vi "ATM_Serv.vi"() -> ()   [LabVIEW 2023]
uses:
  Controller/ControllerATM.ctl
  Controller/ControllerMenu.ctl
  Controller/ControllerAccount.ctl
  <vilib>/Utility/file.llb/Read Delimited Spreadsheet (string).vi
  <vilib>/Utility/file.llb/Write Delimited Spreadsheet (string).vi
  <vilib>/regexp/Match Regular Expression.xnode
panel:
  out "event error":errorcluster
  out "Output":string
  out "login error":errorcluster
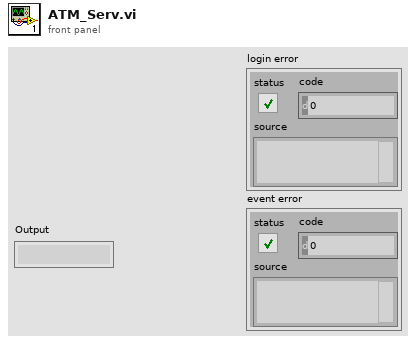
[diagram p1: front panel]
types:
  T1 = typedef "ControllerAccount.ctl" = enum16{"Deactivate", "Deposit", "Withdraw"}
  T2 = typedef "ControllerMenu.ctl" = enum16{"Initialization", "Processes"}
  T3 = typedef "ControllerATM.ctl" = enum16{"Welcome", "Login", "Main"}
  T4 = enum16{"open", "replace", "create", "open or create", "replace or create", "replace or create with confirmation"}
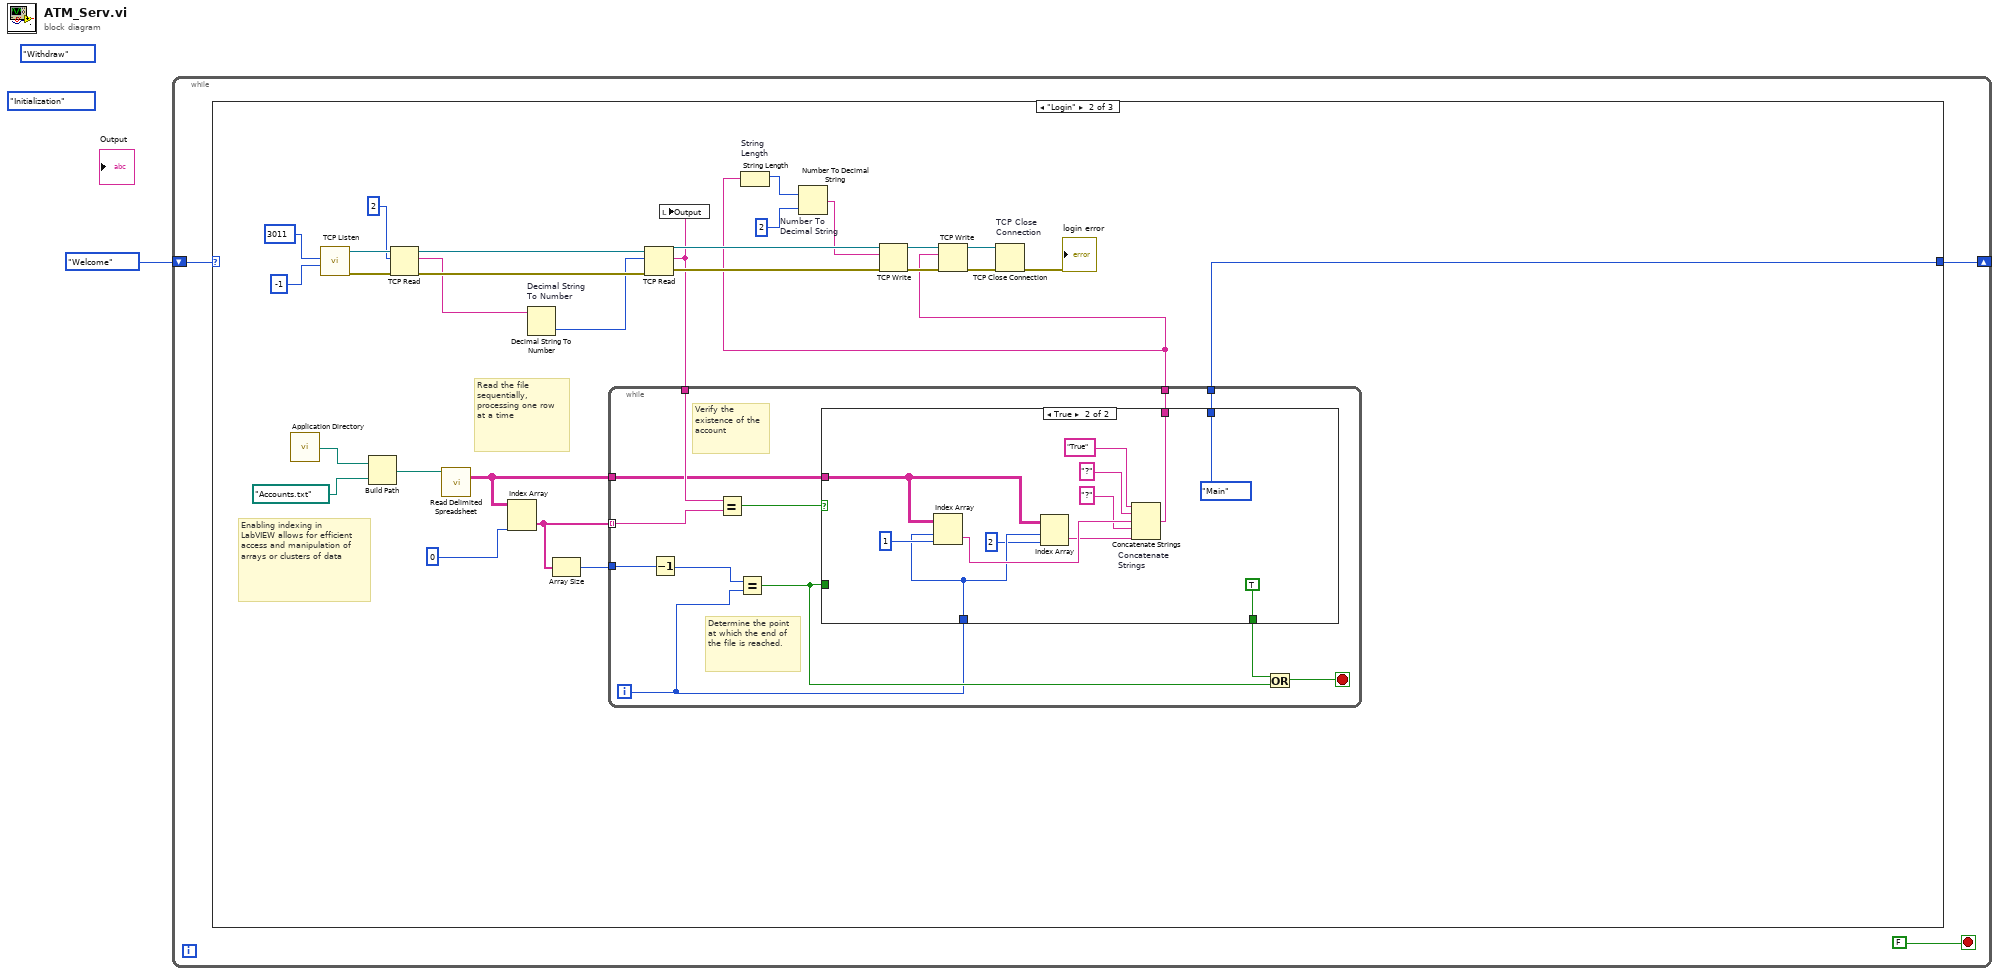
[diagram p0: block diagram]
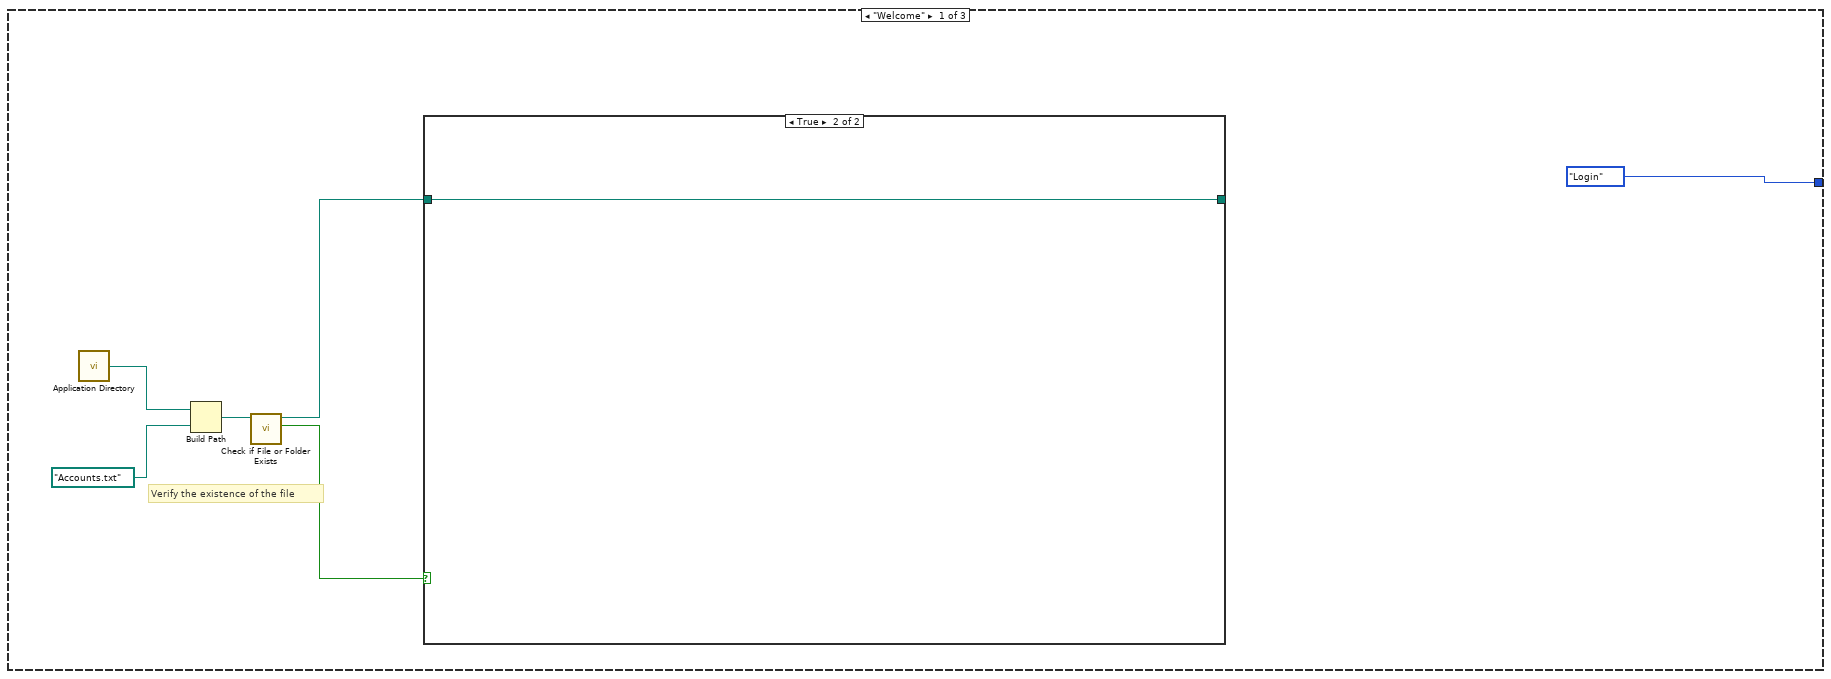
[diagram p2: hidden frame]
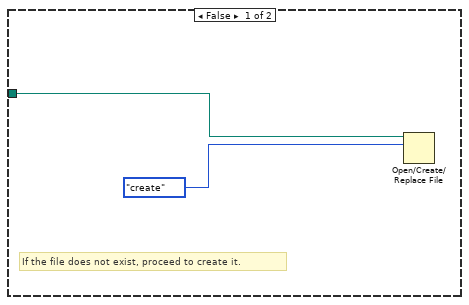
[diagram p3: hidden frame]
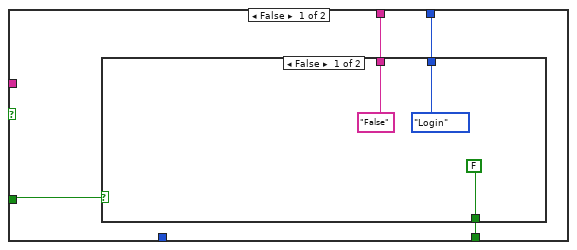
[diagram p4: hidden frame]
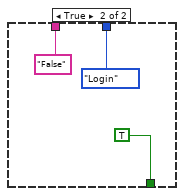
[diagram p5: hidden frame]
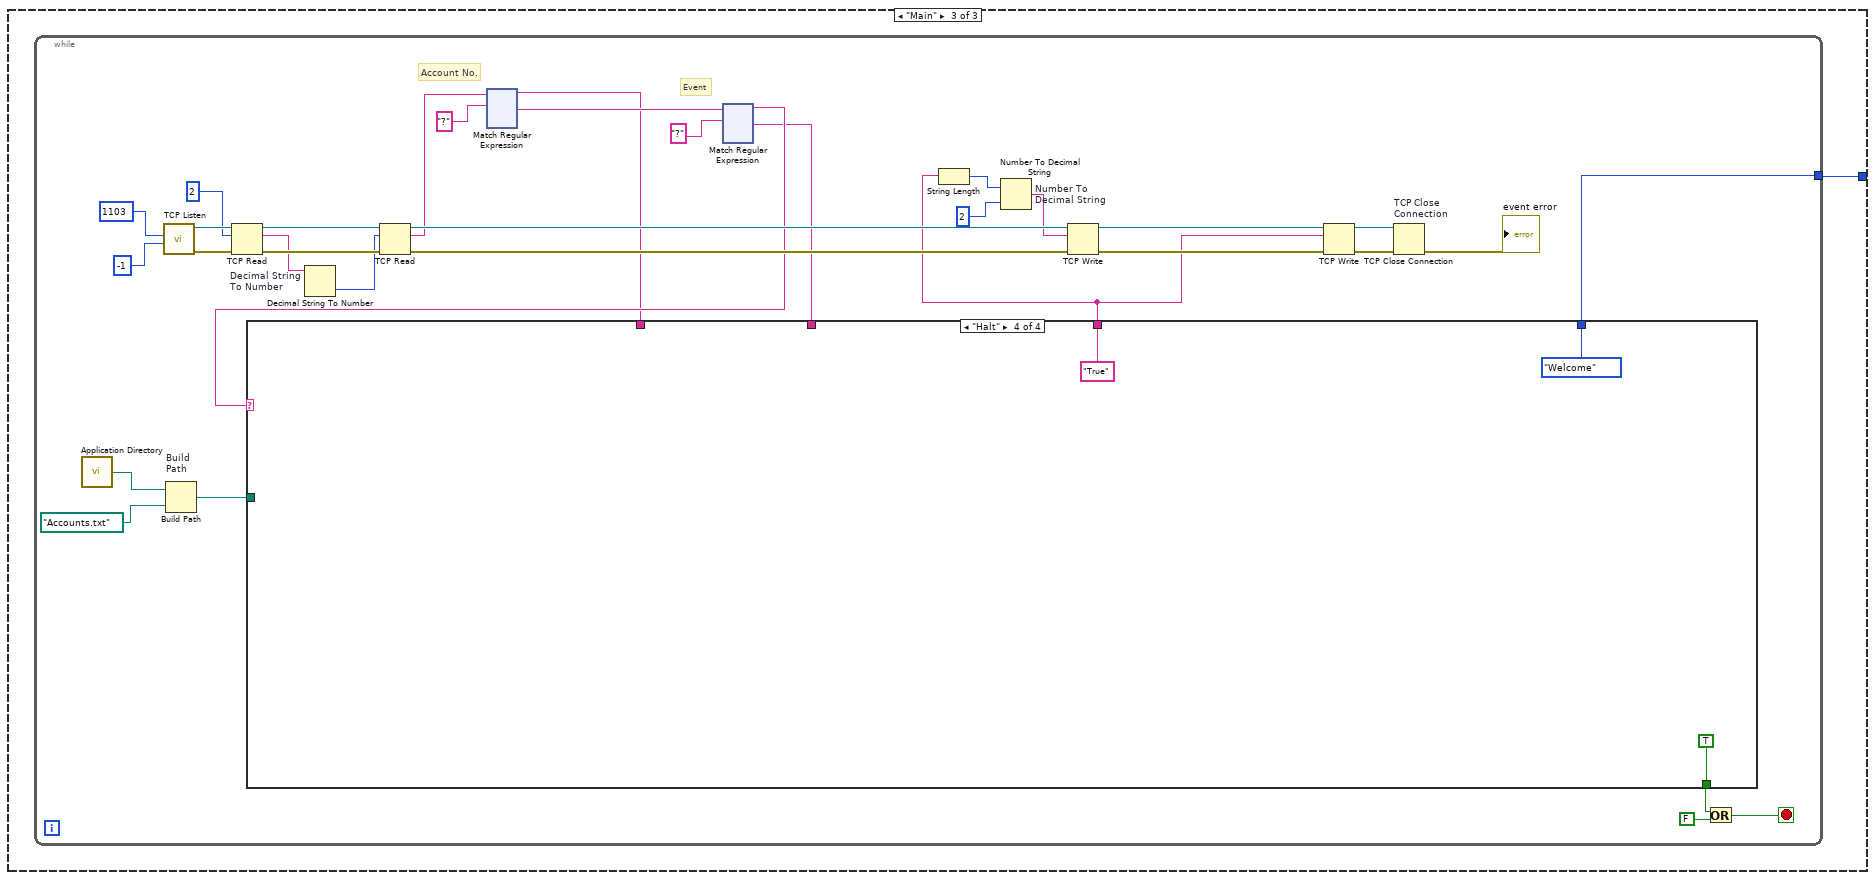
[diagram p6: hidden frame]
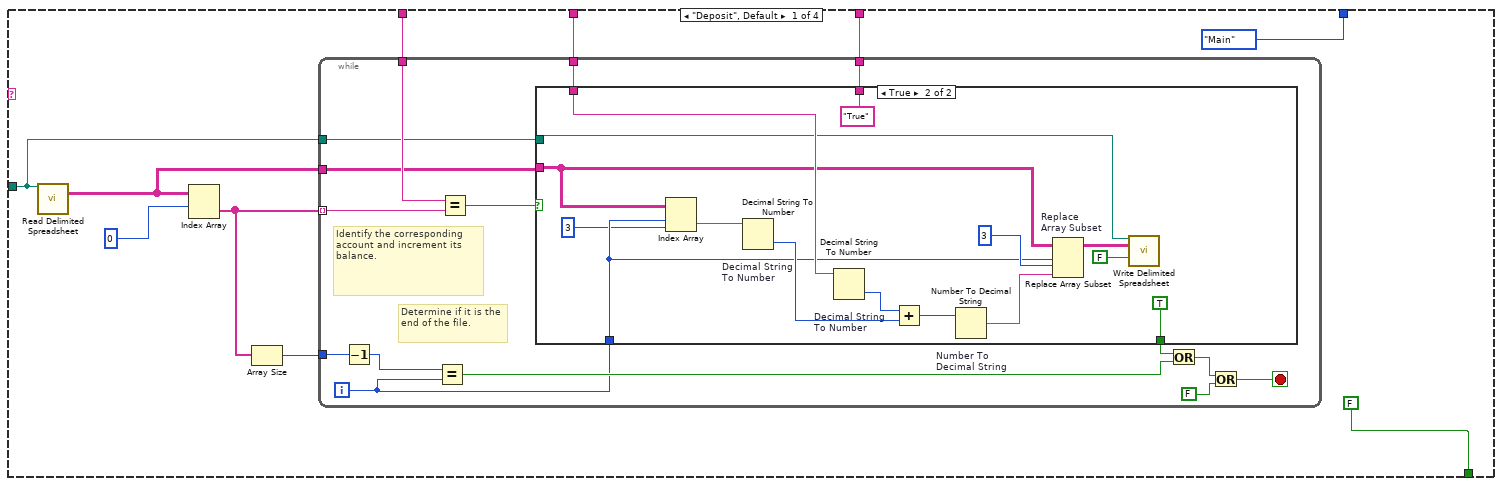
[diagram p7: hidden frame]
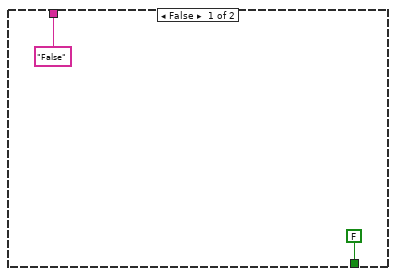
[diagram p8: hidden frame]
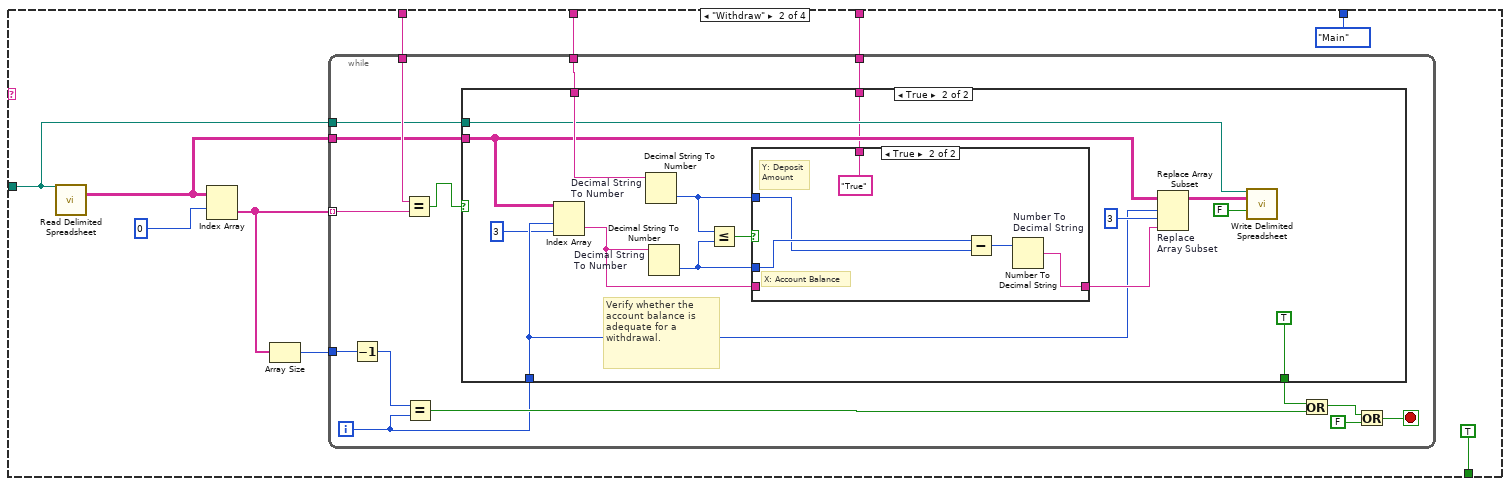
[diagram p9: hidden frame]
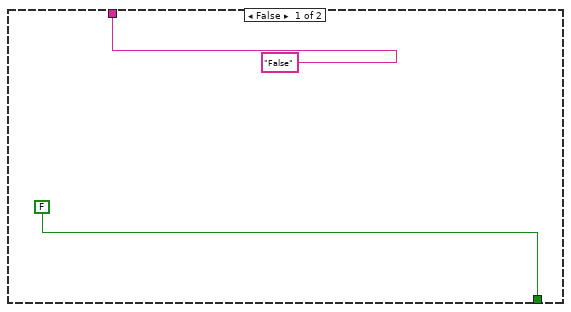
[diagram p10: hidden frame]
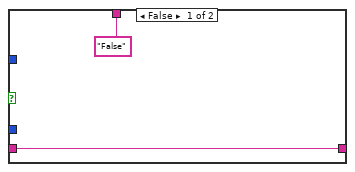
[diagram p11: hidden frame]
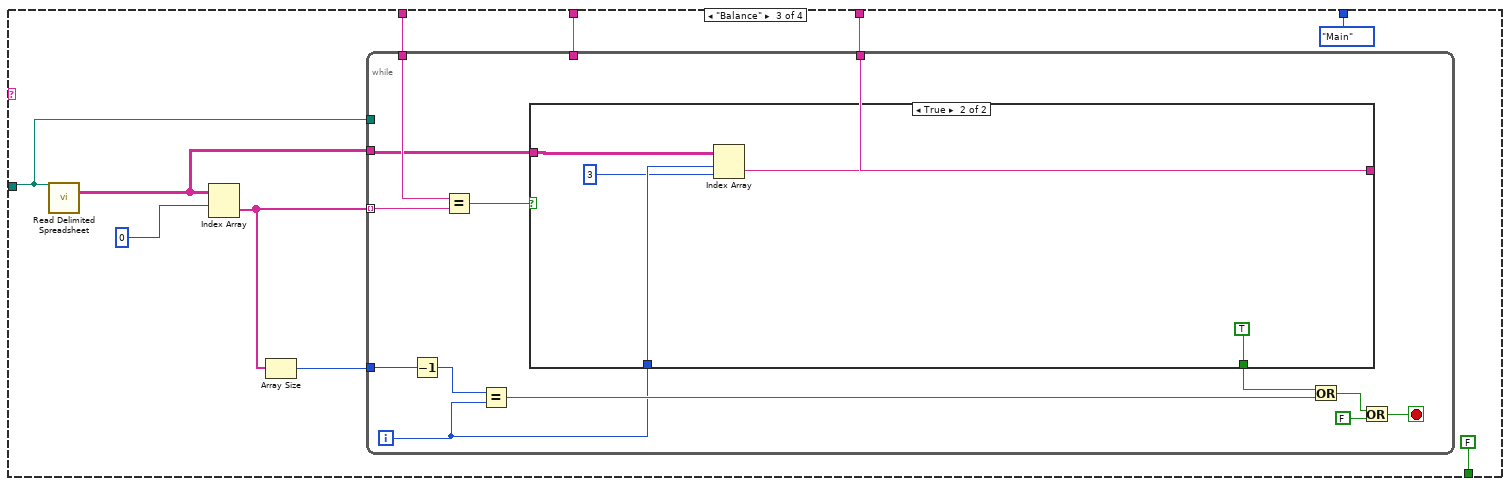
[diagram p12: hidden frame]
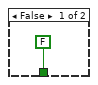
[diagram p13: hidden frame]
diagram:
  (unwired) ControllerAccount."Withdraw" ("Enter")
  (unwired) ControllerMenu."Initialization"
  n1 = while {
    shift-right: [w2] -> _
    shift-left: ControllerATM."Welcome" -> [w3]
    stop <- FALSE stop-if-true
    n2 = case shown="\"Login\"" w3 {
      tunnel: [ControllerATM."Login" w15 w77] -> w2
      frame "Welcome" {
        # "Verify the existence of the file"
        n3 = call <vilib>:"Application Directory.vi"() -> ("Application Directory"=w9:path)
        n4 = Build Path(base path=w9, name or relative path=path "Accounts.txt") -> (appended path=w7:path)
        n5 = call <vilib>:"Check if File or Folder Exists.vi"("path"=w7) -> ("file or folder exists?"=w8:bool, "dup path"=w6:path)  [unwired: 8 in, 1 out]
        n6 = case shown="True" w8 {
          tunnel: w6 -> [w11 w13]
          tunnel: [_ w13] -> _
          frame False {
            # "If the file does not exist, proceed to create it."
            n7 = Open/Create/Replace File(file path (use dialog)=w11, operation (0:open)=T4."create") -> ()  [unwired: 4 in, 3 out]
          }
          frame True {
          }
        }
      }
      frame "Login" {
        # "Enabling indexing in LabVIEW allows for efficient access and manipulation of arrays or clusters of data"
        # "Read the file sequentially, processing one row at a time"
        n8 = call <vilib>:"Application Directory.vi"() -> ("Application Directory"=w22:path)
        n9 = call <vilib>:"TCP Listen.vi"("timeout ms (wait forever: -1)"=-1, "port"=u16 3011) -> ("error out"=w38:errorcluster, "connection ID"=w42:refnum<k5>)  [unwired: 5 in, 3 out]
        n10 = Build Path(base path=w22, name or relative path=path "Accounts.txt") -> (appended path=w23:path)
        n11 = TCP Read(connection ID=w42, bytes to read=2, error in (no error)=w38) -> (connection ID out=w41:refnum<k5>, data out=w29:string, error out=w37:errorcluster)  [unwired: 2 in]
        n12 = call-poly <vilib>:"Read Delimited Spreadsheet.vi"("file path (dialog if empty)"=w23) -> ("all rows"=w20:string[][])  [unwired: 9 in, 5 out]
        n13 = Index Array "Index Array"(array=w20, index (col)=0 ("index (row)")) -> (element=w19:string[])  [unwired: 1 in]
        n14 = Decimal String To Number "Decimal String \nTo Number"(string=w29) -> (number=w28:i32)  [unwired: 2 in, 1 out]
        n15 = Array Size(array=w19) -> (size(s)=w18:i32)
        n16 = TCP Read(connection ID=w41, bytes to read=w28, error in (no error)=w37) -> (connection ID out=w40:refnum<k5>, data out=w24:string, error out=w36:errorcluster)  [unwired: 2 in]
        n17 = while {
          tunnel: w24 -> [w49]
          tunnel: w19 -> [w48] mode=indexing
          tunnel: w20 -> [w46]
          tunnel: w18 -> [w54]
          tunnel: [w44] -> w16
          tunnel: [w43] -> w15
          i -> [w45]
          stop <- w51 stop-if-true
          # "Determine the point at which the end of the file is reached."
          # "Verify the existence of the account"
          n18 = Decrement(x=w54) -> (x-1=w53:i32)
          n19 = Equal?(x=w49, y=w48) -> (x = y?=w47:bool)
          n20 = Equal?(x=w53, y=w45) -> (x = y?=w50:bool)
          n21 = case shown="True" w47 {
            tunnel: w50 -> [w58 _]
            tunnel: [w56 TRUE] -> w52
            tunnel: w46 -> [_ w75]
            tunnel: w45 -> [_ w67]
            tunnel: [w57 w69] -> w44
            tunnel: [w55 ControllerATM."Main"] -> w43
            frame False {
              n22 = case shown="False" w58 {
                tunnel: ["False" "False"] -> w57
                tunnel: [ControllerATM."Login" ControllerATM."Login"] -> w55
                tunnel: [FALSE TRUE] -> w56
                frame False {
                }
                frame True {
                }
              }
            }
            frame True {
              n23 = Index Array "Index Array"(array=w75, index (row)=w67, index (col)=1 ("index (row)")) -> (element=w72:string)
              n24 = Index Array "Index Array"(array=w75, index (row)=w67, index (col)=2 ("index (row)")) -> (element=w70:string)
              n25 = Concatenate Strings "Concatenate\nStrings"("True" ("string"), "?" ("string"), w72, "?" ("string"), w70) -> (w69:string)
            }
          }
          n26 = Or(x=w52, y=w50) -> (x .or. y?=w51:bool)
        }
        n27 = local write "Output"(w24) -> ()
        n28 = String Length "String \nLength"(string=w16) -> (length=w25:i32)
        n29 = Number To Decimal String "Number To \nDecimal String"(number=w25, width (-)=i16 2) -> (decimal integer string=w27:string)
        n30 = TCP Write(connection ID=w40, data in=w27, error in (no error)=w36) -> (connection ID out=w17:refnum<k5>, error out=w35:errorcluster)  [unwired: 1 in, 1 out]
        n31 = TCP Write(connection ID=w17, data in=w16, error in (no error)=w35) -> (connection ID out=w39:refnum<k5>, error out=w34:errorcluster)  [unwired: 1 in, 1 out]
        n32 = TCP Close Connection "TCP Close \nConnection"(connection ID=w39, error in (no error)=w34) -> (error out=→"login error":errorcluster)  [unwired: 1 in, 1 out]
      }
      frame "Main" {
        n33 = while {
          tunnel: [w81] -> w77
          stop <- w80 stop-if-true
          # "Event"
          # "Account No."
          n34 = call <vilib>:"Application Directory.vi"() -> ("Application Directory"=w88:path)
          n35 = call <vilib>:"TCP Listen.vi"("timeout ms (wait forever: -1)"=-1, "port"=u16 1103) -> ("error out"=w106:errorcluster, "connection ID"=w111:refnum<k5>)  [unwired: 5 in, 3 out]
          n36 = Build Path "Build\nPath"(base path=w88, name or relative path=path "Accounts.txt") -> (appended path=w84:path)
          n37 = TCP Read(connection ID=w111, bytes to read=2, error in (no error)=w106) -> (connection ID out=w110:refnum<k5>, data out=w97:string, error out=w105:errorcluster)  [unwired: 2 in]
          n38 = Decimal String To Number "Decimal String\nTo Number"(string=w97) -> (number=w96:i32)  [unwired: 2 in, 1 out]
          n39 = TCP Read(connection ID=w110, bytes to read=w96, error in (no error)=w105) -> (connection ID out=w109:refnum<k5>, data out=w95:string, error out=w104:errorcluster)  [unwired: 2 in]
          n40 = xnode "Match Regular \nExpression"("input string"=w95, "regular expression"="?") -> ("before match"=w85:string, "after match"=w93:string)  [unwired: 4 in, 3 out]
          n41 = xnode "Match Regular \nExpression"("input string"=w93, "regular expression"="?") -> ("before match"=w86:string, "after match"=w83:string)  [unwired: 4 in, 3 out]
          n42 = case shown="\"Halt\"" w86 {
            tunnel: w84 -> [w112 w157 w208 _]
            tunnel: w85 -> [w118 w156 w207 _]
            tunnel: w83 -> [w116 w155 w206 _]
            tunnel: [w115 w154 w205 "True"] -> w82
            tunnel: [ControllerATM."Main" ControllerATM."Main" ControllerATM."Main" ControllerATM."Welcome"] -> w81
            tunnel: [FALSE ("x") TRUE ("x") FALSE ("x") TRUE ("x")] -> w78
            frame "Deposit", Default {
              n43 = call-poly <vilib>:"Read Delimited Spreadsheet.vi"("file path (dialog if empty)"=w112) -> ("all rows"=w117:string[][])  [unwired: 9 in, 5 out]
              n44 = Index Array "Index Array"(array=w117, index (row)=0 ("index")) -> (element=w119:string[])  [unwired: 1 in]
              n45 = Array Size(array=w119) -> (size(s)=w120:i32)
              n46 = while {
                tunnel: w120 -> [w131]
                tunnel: w119 -> [w129] mode=indexing
                tunnel: w118 -> [w128]
                tunnel: w117 -> [w125]
                tunnel: w112 -> [w123]
                tunnel: w116 -> [w124]
                tunnel: [w122] -> w115
                i -> [w126]
                stop <- w136 stop-if-true
                # "Determine if it is the end of the file."
                # "Identify the corresponding account and increment its balance."
                n47 = Decrement(x=w131) -> (x-1=w132:i32)
                n48 = Equal?(x=w132, y=w126) -> (x = y?=w130:bool)
                n49 = Equal?(x=w128, y=w129) -> (x = y?=w127:bool)
                n50 = case shown="True" w127 {
                  tunnel: [FALSE TRUE] -> w133
                  tunnel: w126 -> [_ w140]
                  tunnel: w125 -> [_ w145]
                  tunnel: w124 -> [_ w151]
                  tunnel: w123 -> [_ w146]
                  tunnel: ["False" "True"] -> w122
                  frame False {
                  }
                  frame True {
                    n51 = Index Array "Index Array"(array=w145, index (row)=w140, index (col)=3 ("disabled index (row)")) -> (element=w152:string)
                    n52 = Decimal String To Number "Decimal String\nTo Number"(string=w152) -> (number=w149:i32)  [unwired: 2 in, 1 out]
                    n53 = Decimal String To Number "Decimal String \nTo Number"(string=w151) -> (number=w150:i32)  [unwired: 2 in, 1 out]
                    n54 = Add(x=w150, y=w149) -> (x+y=w148:i32)
                    n55 = Number To Decimal String "Number To \nDecimal String"(number=w148) -> (decimal integer string=w143:string)  [unwired: 1 in]
                    n56 = Replace Array Subset "Replace \nArray Subset"(array=w145, new element=w143, index (row)=w140, index (col)=3 ("disabled index (col)")) -> (w142:string[][])
                    n57 = call-poly <vilib>:"Write Delimited Spreadsheet.vi"("file path (dialog if empty)"=w146, "2D data"=w142, "append to file? (new file:F)"=FALSE) -> ()  [unwired: 11 in, 2 out]
                  }
                }
                n58 = Or(x=w133, y=w130) -> (x .or. y?=w134:bool)
                n59 = Or(x=w134, y=FALSE) -> (x .or. y?=w136:bool)
              }
            }
            frame "Withdraw" {
              n60 = call-poly <vilib>:"Read Delimited Spreadsheet.vi"("file path (dialog if empty)"=w157) -> ("all rows"=w158:string[][])  [unwired: 9 in, 5 out]
              n61 = Index Array "Index Array"(array=w158, index (row)=0 ("index")) -> (element=w159:string[])  [unwired: 1 in]
              n62 = Array Size(array=w159) -> (size(s)=w160:i32)
              n63 = while {
                tunnel: w160 -> [w176]
                tunnel: w159 -> [w172] mode=indexing
                tunnel: w158 -> [w168]
                tunnel: w157 -> [w167]
                tunnel: w156 -> [w171]
                tunnel: w155 -> [w166]
                tunnel: [w165] -> w154
                i -> [w170]
                stop <- w178 stop-if-true
                n64 = Decrement(x=w176) -> (x-1=w177:i32)
                n65 = Equal?(x=w171, y=w172) -> (x = y?=w169:bool)
                n66 = Equal?(x=w177, y=w170) -> (x = y?=w173:bool)
                n67 = case shown="True" w169 {
                  tunnel: [FALSE TRUE] -> w164
                  tunnel: w170 -> [_ w182]
                  tunnel: w168 -> [_ w191]
                  tunnel: w166 -> [_ w194]
                  tunnel: w167 -> [_ w192]
                  tunnel: ["False" w184] -> w165
                  frame False {
                  }
                  frame True {
                    # "Verify whether the account balance is adequate for a withdrawal."
                    n68 = Index Array "Index Array"(array=w191, index (row)=w182, index (col)=3 ("disabled index (row)")) -> (element=w183:string)
                    n69 = Decimal String To Number "Decimal String\nTo Number"(string=w194) -> (number=w187:i32)  [unwired: 2 in, 1 out]
                    n70 = Decimal String To Number "Decimal String\nTo Number"(string=w183) -> (number=w186:i32)  [unwired: 2 in, 1 out]
                    n71 = Less Or Equal?(x=w187, y=w186) -> (x <= y?=w188:bool)
                    n72 = case shown="True" w188 {
                      tunnel: w187 -> [_ w198]
                      tunnel: w186 -> [_ w199]
                      tunnel: [w196 w202] -> w185
                      tunnel: ["False" "True"] -> w184
                      tunnel: w183 -> [w196 _]
                      frame False {
                      }
                      frame True {
                        # "Y: Deposit \nAmount"
                        # "X: Account Balance"
                        n73 = Subtract(x=w199, y=w198) -> (x-y=w201:i32)
                        n74 = Number To Decimal String "Number To\nDecimal String"(number=w201) -> (decimal integer string=w202:string)  [unwired: 1 in]
                      }
                    }
                    n75 = Replace Array Subset "Replace \nArray Subset"(array=w191, new element=w185, index (row)=w182, index (col)=3 ("disabled index (col)")) -> (w189:string[][])
                    n76 = call-poly <vilib>:"Write Delimited Spreadsheet.vi"("file path (dialog if empty)"=w192, "2D data"=w189, "append to file? (new file:F)"=FALSE) -> ()  [unwired: 11 in, 2 out]
                  }
                }
                n77 = Or(x=w164, y=w173) -> (x .or. y?=w174:bool)
                n78 = Or(x=w174, y=FALSE) -> (x .or. y?=w178:bool)
              }
            }
            frame "Balance" {
              n79 = call-poly <vilib>:"Read Delimited Spreadsheet.vi"("file path (dialog if empty)"=w208) -> ("all rows"=w209:string[][])  [unwired: 9 in, 5 out]
              n80 = Index Array "Index Array"(array=w209, index (row)=0 ("index")) -> (element=w210:string[])  [unwired: 1 in]
              n81 = Array Size(array=w210) -> (size(s)=w211:i32)
              n82 = while {
                tunnel: w211 -> [w223]
                tunnel: w210 -> [w221] mode=indexing
                tunnel: w209 -> [w219]
                tunnel: w208 -> [_]
                tunnel: w207 -> [w220]
                tunnel: w206 -> [_]
                tunnel: [w213] -> w205
                i -> [w214]
                stop <- w225 stop-if-true
                n83 = Decrement(x=w223) -> (x-1=w224:i32)
                n84 = Equal?(x=w220, y=w221) -> (x = y?=w218:bool)
                n85 = Equal?(x=w224, y=w214) -> (x = y?=w216:bool)
                n86 = case shown="True" w218 {
                  tunnel: w219 -> [_ w230]
                  tunnel: [FALSE TRUE ("x")] -> w215
                  tunnel: w214 -> [_ w229]
                  tunnel: [_ w227] -> w213
                  frame False {
                  }
                  frame True {
                    n87 = Index Array "Index Array"(array=w230, index (row)=w229, index (col)=3 ("disabled index (col)")) -> (element=w227:string)
                  }
                }
                n88 = Or(x=w215, y=w216) -> (x .or. y?=w217:bool)
                n89 = Or(x=w217, y=FALSE) -> (x .or. y?=w225:bool)
              }
            }
            frame "Halt" {
            }
          }
          n90 = String Length(string=w82) -> (length=w90:i32)
          n91 = Number To Decimal String "Number To\nDecimal String"(number=w90, width (-)=i16 2) -> (decimal integer string=w89:string)
          n92 = TCP Write(connection ID=w109, data in=w89, error in (no error)=w104) -> (connection ID out=w108:refnum<k5>, error out=w103:errorcluster)  [unwired: 1 in, 1 out]
          n93 = TCP Write(connection ID=w108, data in=w82, error in (no error)=w103) -> (connection ID out=w107:refnum<k5>, error out=w102:errorcluster)  [unwired: 1 in, 1 out]
          n94 = TCP Close Connection "TCP Close \nConnection"(connection ID=w107, error in (no error)=w102) -> (error out=→"event error":errorcluster)  [unwired: 1 in, 1 out]
          n95 = Or(x=w78, y=FALSE) -> (x .or. y?=w80:bool)
        }
      }
    }
  }
